vi "AuMT8852B Single-slot Sensitivity Configuration.vi"(5 "Settings":T1={"Low frequency selection"=enum."Use low frequency", "Medium frequency selection"=enum."Use medium frequency", "High frequency selection"=enum."Use high frequency", "Low TX frequency"=2480.0, "Low RX frequency"=2402.0, "Medium TX frequency"=2402.0, "Medium RX frequency"=2441.0, "High TX frequency"=2402.0, "High RX frequency"=2480.0, "Number of packets"=7408, "Test TX power"=-70.0, "BER limit"=0.1, "FER limit"=100.0, "Hop selection"=enum."Test with hopping off and on", "Packet count"=enum."TX", "Use Dirty transmitter"=FALSE, "Frequency offset (kHz)"=[75.0, 14.0, -2.0, 1.0, 39.0, 0.0, -42.0, 74.0, -19.0, -75.0], "Symbol timing error (ppm)"=[-20.0, -20.0, 20.0, 20.0, 20.0, -20.0, -20.0, -20.0, -20.0, 20.0], "Modulation index"=[0.28, 0.3, 0.29, 0.32, 0.33, 0.34, 0.29, 0.31, 0.28, 0.35]} {"Frequency offset (kHz)" format="%.2f"; "Symbol timing error (ppm)" format="%.2f"; "FER limit" format="%.2f"; "BER limit" format="%.2f"; "Modulation index" format="%.2f"; "Test TX power" format="%.1f"}, 7 "Set/Get (Set)":enum16{"Set", "Get"}(ring), 8 "error in (no error)":errorcluster, 10 "Script (3)":i32=3, 11 "VISA session":refnum<visa-resource-name>) -> (0 "error out":errorcluster, 2 "error code":i32, 3 "VISA session out":refnum<visa-resource-name>, 4 "Settings out":T1={"Low frequency selection"=enum."Use low frequency", "Medium frequency selection"=enum."Use medium frequency", "High frequency selection"=enum."Use high frequency", "Low TX frequency"=0.0, "Low RX frequency"=0.0, "Medium TX frequency"=0.0, "Medium RX frequency"=0.0, "High TX frequency"=0.0, "High RX frequency"=0.0, "Number of packets"=0, "Test TX power"=0.0, "BER limit"=0.0, "FER limit"=0.0, "Hop selection"=enum."Test with hopping on", "Packet count"=enum."TX", "Use Dirty transmitter"=FALSE, "Frequency offset (kHz)"=[], "Symbol timing error (ppm)"=[], "Modulation index"=[]} {"Symbol timing error (ppm)" format="%.2f"; "Modulation index" format="%.2f"; "Frequency offset (kHz)" format="%.2f"; "FER limit" format="%.2f"; "BER limit" format="%.2f"; "Test TX power" format="%.1f"})   [LabVIEW 2017]
doc: "Anritsu MT8852B Bluetooth Tester\n\nConfigures the instrument for the Single-slot Sensitivity test.\n\nINPUTS\nSet/Get - whether the values are being sent to or retrieved from the instrument.\nScript - which of the stored scripts (1-10) will be queried or configured. Scripts 1 and 2 are read-only.\nSettings - parameters of the test to be written.\n\nOUTPUTS\nSettings out - current parameters of the test."
uses:
  <instrlib>/aumt8852B/General/Utilities/MT8850 Test Parameters.ctl
  <instrlib>/aumt8852B/General/Utilities/MT8850 Frequency Units.ctl
panel:
  in  "Case Constant\n(See Context Help)":bool
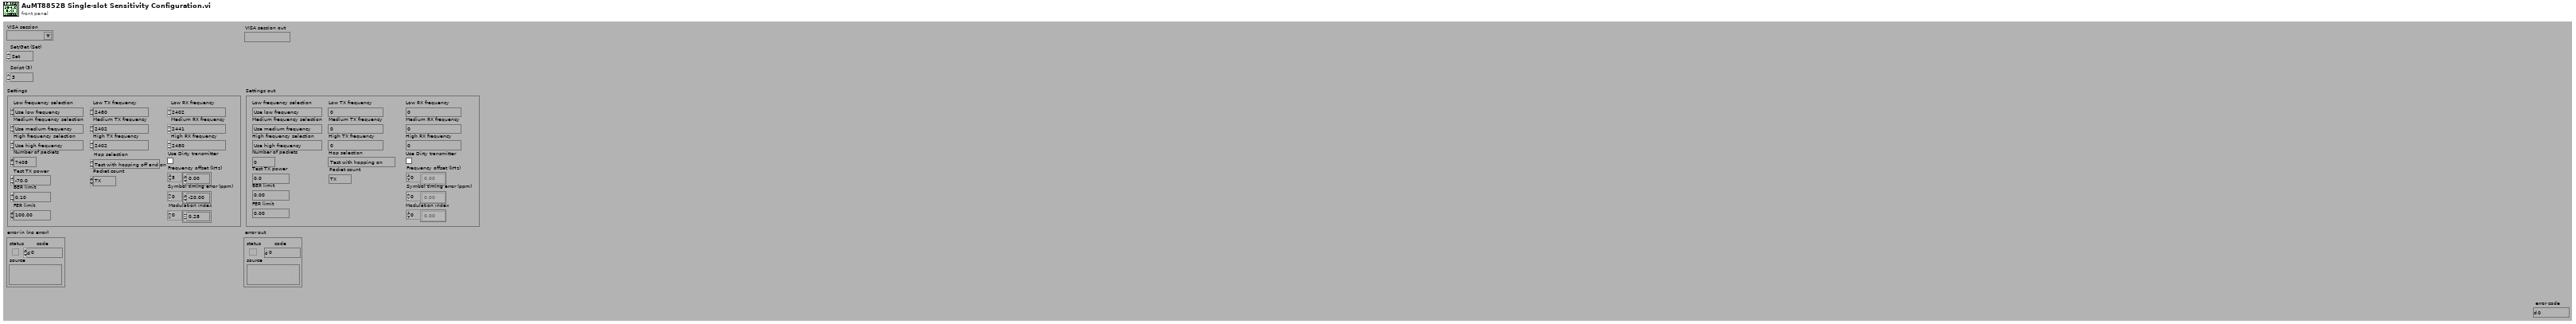
[diagram p1: front panel]
types:
  T1 = cluster{"Low frequency selection":enum16{"Don't use low frequency", "Use low frequency"}, "Medium frequency selection":enum16{"Don't use medium frequency", "Use medium frequency"}, "High frequency selection":enum16{"Don't use high frequency", "Use high frequency"}, "Low TX frequency":dbl, "Low RX frequency":dbl, "Medium TX frequency":dbl, "Medium RX frequency":dbl, "High TX frequency":dbl, "High RX frequency":dbl, "Number of packets":i32, "Test TX power":dbl, "BER limit":dbl, "FER limit":dbl, "Hop selection":enum16{"Test with hopping on", "Test with hopping off", "Test with hopping off and on"}, "Packet count":enum16{"TX", "RX"}, "Use Dirty transmitter":bool, "Frequency offset (kHz)":dbl[], "Symbol timing error (ppm)":dbl[], "Modulation index":dbl[]}
  T2 = typedef "MT8850 Test Parameters.ctl" = enum16{"Use low frequency", "Use medium frequency", "Use high frequency", "Low TX frequency", "Low RX frquency", "Medium TX frequency", "Medium RX frequency", "High TX frequency", "High RX frequency", "Number of packets", "Average high limit", "Average low limit", "Peak power limit", "Max power step limit", "Min power step limit", "f1 average minimum", "f1 average maximum", "f2 maximum", "f1/f2 average maximum", "Hop selection", "Use DH1 packets", "Use DH3 packets", "Use DH5 packets", "1 slot packet drift limit", "3 slot packet drift limit", "5 slot packet drift limit", "Drift rate limit", "TX power level", "Frequency offset", "Symbol timing", "Modulation index", "BER limit", "FER limit", "Use averaging high limit", "Use averaging low limit", "Use peak power limit", "Packet type", "Test control", "Use max power step limit", "Use min power step limit", "Number of cycles", "Use f1 average maximum", "Use f1 average minimum", "Use f2 maximum", "Use f1/f2 average maximum", "Hop mode", "Maximum negative limit", "Maximum positive limit", "Use maximum negative limit", "Use maximum positive limit", "Use 1 slot packet drift limit", "Use 3 slot packet drift limit", "Use 5 slot packet drift limit", "Use drift rate limit", "Use BER limit", "Use FER limit", "Use dirty parameter table", "Use null packet drift limit", "Null packet drift limit", "Minimum power", "Power delay", "Packet count", "Payload toggle", "Output power level", "2DHX packet type", "3DHX packet type", "Number of blocks", "TX and RX low frequency", "TX and RX medium frequency", "TX and RX high frequency", "TX frequency", "RX frequency", "Threshold bit count", "Total test bit count", "Number of bits", "PDPSK to PGFSK lower limit", "PDPSK to PGFSK upper limit", "Initial frequency error upper limit", "Initial frequency error lower limit", "Frequency error upper limit", "Frequency error lower limit", "Block frequency error upper limit", "Block frequency error lower limit", "2Mbs RMS DEVM limit", "3Mbs RMS DEVM limit", "2Mbs Peak DEVM limit", "3Mbs Peak DEVM limit", "2Mbs 99% packets DEVM limit", "3Mbs 99% packets DEVM limit", "Percentage of no error packets limit", "Threshold error limit", "Total test error limit"}
  T3 = enum16{"Single-slot sensitivity", "Multiple-slot sensitivity"}
  T4 = enum16{"Frequency offset", "Symbol timing value", "Mod index value"}
  T5 = typedef "MT8850 Frequency Units.ctl" = enum16{"Channel", "Hz", "kHz", "MHz", "GHz"}
  T6 = enum16{"Simulate", "Range check", "Cache", "Query instrument status"}
  T7 = enum16{"Output power", "Power control", "Modulation characteristics", "Initial carrier", "Carrier drift", "Single slot sensitivity", "Multiple slot sensitivity", "Maximum input power"}
  T8 = enum16{"Test with hopping on", "Test with hopping off", "Test with hopping off and on"}
  T9 = enum16{"Don't use high frequency", "Use high frequency"}
  T10 = enum16{"Don't use medium frequency", "Use medium frequency"}
  T11 = enum16{"Don't use low frequency", "Use low frequency"}
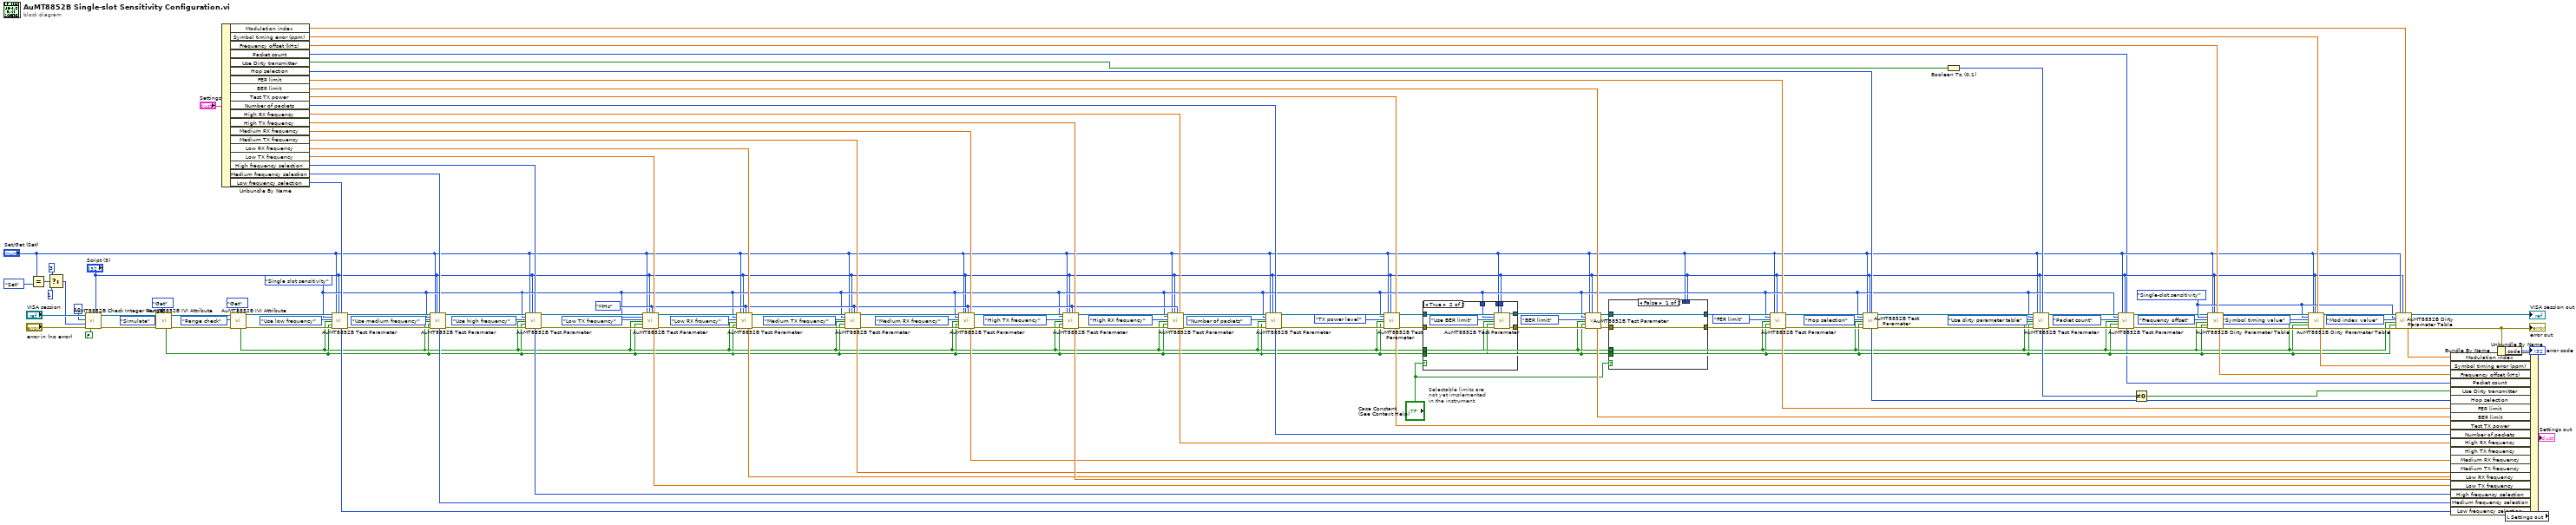
[diagram p0: block diagram]
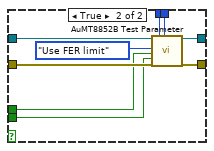
[diagram p2: hidden frame]
diagram:
  w13 = T3."Single-slot sensitivity" ("Test (Single-slot sensitivity)")
  w35 = MT8850_Frequency_Units."MHz" ("Frequency units (MHz)")
  w8 = T7."Single slot sensitivity" ("Test (Output Power)")
  # "Selectable limits are\nnot yet implemented\nin the instrument."
  n1 = Equal?(x="Set/Get (Set)", y=enum16{"Set", "Get"}."Set") -> (x = y?=w129:bool)
  n2 = Select(t=3, s=w129, f=1) -> (s? t:f=w125:i32)
  n3 = call <instrlib>:"AuMT8852B Check Integer Range.vi"("Value (0)"="Script (3)", "Check IVI flag first? (T)"=FALSE, "error in (no error)"="error in (no error)", "Lower limit (-1)"=w125, "Upper limit (1)"=10, "VISA session"="VISA session") -> ("error out"=w123:errorcluster, "VISA session out"=w124:refnum<visa-resource-name>)  [unwired: 4 in]
  n4 = call <instrlib>:"AuMT8852B IVI Attribute.vi"("Set/Get (Set)"=enum16{"Set", "Get"}."Get", "error in (no error)"=w123, "Flag (Simulate)"=T6."Simulate", "VISA session"=w124) -> ("error out"=w97:errorcluster, "VISA session out"=w98:refnum<visa-resource-name>, "Value out"=w3:bool)  [unwired: 5 in]
  n5 = Unbundle By Name("Settings") -> ("Modulation index"=w24:dbl[], "Symbol timing error (ppm)"=w25:dbl[], "Frequency offset (kHz)"=w29:dbl[], "Packet count"=w1:enum16{"TX", "RX"}, "Use Dirty transmitter"=w47:bool, "Hop selection"=w51:T8, "FER limit"=w65:dbl, "BER limit"=w66:dbl, "Test TX power"=w70:dbl, "Number of packets"=w71:i32, "High RX frequency"=w84:dbl, "High TX frequency"=w85:dbl, "Medium RX frequency"=w72:dbl, "Medium TX frequency"=w86:dbl, "Low RX frequency"=w87:dbl, "Low TX frequency"=w88:dbl, "High frequency selection"=w89:T9, "Medium frequency selection"=w90:T10, "Low frequency selection"=w91:T11)
  n6 = call <instrlib>:"AuMT8852B IVI Attribute.vi"("Set/Get (Set)"=enum16{"Set", "Get"}."Get", "error in (no error)"=w97, "Flag (Simulate)"=T6."Range check", "VISA session"=w98) -> ("error out"=w95:errorcluster, "VISA session out"=w96:refnum<visa-resource-name>, "Value out"=w4:bool)  [unwired: 5 in]
  n7 = call <instrlib>:"AuMT8852B Test Parameter.vi"("VISA session"=w96, "Test (Output power)"=w8, "Parameter (Use low frequency)"=MT8850_Test_Parameters."Use low frequency", "Range check? (F)"=w4, "Simulate? (F)"=w3, "error in (no error)"=w95, "Set/Get (Set)"="Set/Get (Set)", "Script (3)"="Script (3)", "Integer value (0)"=w91) -> ("Integer value out"=w76:i32, "VISA session out"=w43:refnum<visa-resource-name>, "error out"=w42:errorcluster)  [unwired: 7 in, 1 out]
  n8 = call <instrlib>:"AuMT8852B Test Parameter.vi"("VISA session"=w43, "Test (Output power)"=w8, "Parameter (Use low frequency)"=MT8850_Test_Parameters."Use medium frequency", "Range check? (F)"=w4, "Simulate? (F)"=w3, "error in (no error)"=w42, "Set/Get (Set)"="Set/Get (Set)", "Script (3)"="Script (3)", "Integer value (0)"=w90) -> ("Integer value out"=w77:i32, "VISA session out"=w41:refnum<visa-resource-name>, "error out"=w40:errorcluster)  [unwired: 7 in, 1 out]
  n9 = call <instrlib>:"AuMT8852B Test Parameter.vi"("VISA session"=w41, "Test (Output power)"=w8, "Parameter (Use low frequency)"=MT8850_Test_Parameters."Use high frequency", "Range check? (F)"=w4, "Simulate? (F)"=w3, "error in (no error)"=w40, "Set/Get (Set)"="Set/Get (Set)", "Script (3)"="Script (3)", "Integer value (0)"=w89) -> ("Integer value out"=w78:i32, "VISA session out"=w119:refnum<visa-resource-name>, "error out"=w118:errorcluster)  [unwired: 7 in, 1 out]
  n10 = call <instrlib>:"AuMT8852B Test Parameter.vi"("VISA session"=w119, "Test (Output power)"=w8, "Parameter (Use low frequency)"=MT8850_Test_Parameters."Low TX frequency", "Range check? (F)"=w4, "Simulate? (F)"=w3, "error in (no error)"=w118, "Set/Get (Set)"="Set/Get (Set)", "Script (3)"="Script (3)", "Integer value (0)"=w35, "Float value (0)"=w88) -> ("Float value out"=w79:dbl, "VISA session out"=w117:refnum<visa-resource-name>, "error out"=w116:errorcluster)  [unwired: 6 in, 1 out]
  n11 = call <instrlib>:"AuMT8852B Test Parameter.vi"("VISA session"=w117, "Test (Output power)"=w8, "Parameter (Use low frequency)"=MT8850_Test_Parameters."Low RX frquency", "Range check? (F)"=w4, "Simulate? (F)"=w3, "error in (no error)"=w116, "Set/Get (Set)"="Set/Get (Set)", "Script (3)"="Script (3)", "Integer value (0)"=w35, "Float value (0)"=w87) -> ("Float value out"=w80:dbl, "VISA session out"=w115:refnum<visa-resource-name>, "error out"=w114:errorcluster)  [unwired: 6 in, 1 out]
  n12 = call <instrlib>:"AuMT8852B Test Parameter.vi"("VISA session"=w115, "Test (Output power)"=w8, "Parameter (Use low frequency)"=MT8850_Test_Parameters."Medium TX frequency", "Range check? (F)"=w4, "Simulate? (F)"=w3, "error in (no error)"=w114, "Set/Get (Set)"="Set/Get (Set)", "Script (3)"="Script (3)", "Integer value (0)"=w35, "Float value (0)"=w86) -> ("Float value out"=w81:dbl, "VISA session out"=w113:refnum<visa-resource-name>, "error out"=w112:errorcluster)  [unwired: 6 in, 1 out]
  n13 = call <instrlib>:"AuMT8852B Test Parameter.vi"("VISA session"=w113, "Test (Output power)"=w8, "Parameter (Use low frequency)"=MT8850_Test_Parameters."Medium RX frequency", "Range check? (F)"=w4, "Simulate? (F)"=w3, "error in (no error)"=w112, "Set/Get (Set)"="Set/Get (Set)", "Script (3)"="Script (3)", "Integer value (0)"=w35, "Float value (0)"=w72) -> ("Float value out"=w74:dbl, "VISA session out"=w111:refnum<visa-resource-name>, "error out"=w110:errorcluster)  [unwired: 6 in, 1 out]
  n14 = call <instrlib>:"AuMT8852B Test Parameter.vi"("VISA session"=w111, "Test (Output power)"=w8, "Parameter (Use low frequency)"=MT8850_Test_Parameters."High TX frequency", "Range check? (F)"=w4, "Simulate? (F)"=w3, "error in (no error)"=w110, "Set/Get (Set)"="Set/Get (Set)", "Script (3)"="Script (3)", "Integer value (0)"=w35, "Float value (0)"=w85) -> ("Float value out"=w82:dbl, "VISA session out"=w109:refnum<visa-resource-name>, "error out"=w108:errorcluster)  [unwired: 6 in, 1 out]
  n15 = call <instrlib>:"AuMT8852B Test Parameter.vi"("VISA session"=w109, "Test (Output power)"=w8, "Parameter (Use low frequency)"=MT8850_Test_Parameters."High RX frequency", "Range check? (F)"=w4, "Simulate? (F)"=w3, "error in (no error)"=w108, "Set/Get (Set)"="Set/Get (Set)", "Script (3)"="Script (3)", "Integer value (0)"=w35, "Float value (0)"=w84) -> ("Float value out"=w83:dbl, "VISA session out"=w107:refnum<visa-resource-name>, "error out"=w106:errorcluster)  [unwired: 6 in, 1 out]
  n16 = call <instrlib>:"AuMT8852B Test Parameter.vi"("VISA session"=w107, "Test (Output power)"=w8, "Parameter (Use low frequency)"=MT8850_Test_Parameters."Number of packets", "Range check? (F)"=w4, "Simulate? (F)"=w3, "error in (no error)"=w106, "Set/Get (Set)"="Set/Get (Set)", "Script (3)"="Script (3)", "Integer value (0)"=w71) -> ("Integer value out"=w73:i32, "VISA session out"=w34:refnum<visa-resource-name>, "error out"=w33:errorcluster)  [unwired: 7 in, 1 out]
  n17 = call <instrlib>:"AuMT8852B Test Parameter.vi"("VISA session"=w34, "Test (Output power)"=w8, "Parameter (Use low frequency)"=MT8850_Test_Parameters."TX power level", "Range check? (F)"=w4, "Simulate? (F)"=w3, "error in (no error)"=w33, "Set/Get (Set)"="Set/Get (Set)", "Script (3)"="Script (3)", "Float value (0)"=w70) -> ("Float value out"=w64:dbl, "VISA session out"=w22:refnum<visa-resource-name>, "error out"=w23:errorcluster)  [unwired: 7 in, 1 out]
  n18 = case shown="True" "Case Constant\n(See Context Help)" {
    tunnel: w23 -> [w133 w143]
    tunnel: w22 -> [w134 w142]
    tunnel: [w134 w141] -> w57
    tunnel: [w133 w140] -> w56
    tunnel: w8 -> [_ w139]
    tunnel: w4 -> [_ w138]
    tunnel: w3 -> [_ w137]
    tunnel: "Set/Get (Set)" -> [_ w136]
    tunnel: "Script (3)" -> [_ w135]
    frame False {
    }
    frame True {
      n19 = call <instrlib>:"AuMT8852B Test Parameter.vi"("VISA session"=w142, "Test (Output power)"=w139, "Parameter (Use low frequency)"=MT8850_Test_Parameters."Use BER limit", "Range check? (F)"=w138, "Simulate? (F)"=w137, "error in (no error)"=w143, "Set/Get (Set)"=w136, "Script (3)"=w135) -> ("VISA session out"=w141:refnum<visa-resource-name>, "error out"=w140:errorcluster)  [unwired: 8 in, 2 out]
    }
  }
  n20 = call <instrlib>:"AuMT8852B Test Parameter.vi"("VISA session"=w57, "Test (Output power)"=w8, "Parameter (Use low frequency)"=MT8850_Test_Parameters."BER limit", "Range check? (F)"=w4, "Simulate? (F)"=w3, "error in (no error)"=w56, "Set/Get (Set)"="Set/Get (Set)", "Script (3)"="Script (3)", "Float value (0)"=w66) -> ("Float value out"=w63:dbl, "VISA session out"=w54:refnum<visa-resource-name>, "error out"=w55:errorcluster)  [unwired: 7 in, 1 out]
  n21 = case shown="False" "Case Constant\n(See Context Help)" {
    tunnel: w55 -> [w145 w154]
    tunnel: w54 -> [w146 w153]
    tunnel: [w146 w152] -> w53
    tunnel: [w145 w151] -> w52
    tunnel: w4 -> [_ w150]
    tunnel: w3 -> [_ w149]
    tunnel: "Set/Get (Set)" -> [_ w148]
    tunnel: "Script (3)" -> [_ w147]
    frame False {
    }
    frame True {
      n22 = call <instrlib>:"AuMT8852B Test Parameter.vi"("VISA session"=w153, "Parameter (Use low frequency)"=MT8850_Test_Parameters."Use FER limit", "Range check? (F)"=w150, "Simulate? (F)"=w149, "error in (no error)"=w154, "Set/Get (Set)"=w148, "Script (3)"=w147) -> ("VISA session out"=w152:refnum<visa-resource-name>, "error out"=w151:errorcluster)  [unwired: 9 in, 2 out]
    }
  }
  n23 = call <instrlib>:"AuMT8852B Test Parameter.vi"("VISA session"=w53, "Test (Output power)"=w8, "Parameter (Use low frequency)"=MT8850_Test_Parameters."FER limit", "Range check? (F)"=w4, "Simulate? (F)"=w3, "error in (no error)"=w52, "Set/Get (Set)"="Set/Get (Set)", "Script (3)"="Script (3)", "Float value (0)"=w65) -> ("Float value out"=w62:dbl, "VISA session out"=w59:refnum<visa-resource-name>, "error out"=w60:errorcluster)  [unwired: 7 in, 1 out]
  n24 = call <instrlib>:"AuMT8852B Test Parameter.vi"("VISA session"=w59, "Test (Output power)"=w8, "Parameter (Use low frequency)"=MT8850_Test_Parameters."Hop selection", "Range check? (F)"=w4, "Simulate? (F)"=w3, "error in (no error)"=w60, "Set/Get (Set)"="Set/Get (Set)", "Script (3)"="Script (3)", "Integer value (0)"=w51) -> ("Integer value out"=w58:i32, "VISA session out"=w32:refnum<visa-resource-name>, "error out"=w31:errorcluster)  [unwired: 7 in, 1 out]
  n25 = Boolean To (0,1)(Boolean=w47) -> (0, 1=w48:i16)
  n26 = call <instrlib>:"AuMT8852B Test Parameter.vi"("VISA session"=w32, "Test (Output power)"=w8, "Parameter (Use low frequency)"=MT8850_Test_Parameters."Use dirty parameter table", "Range check? (F)"=w4, "Simulate? (F)"=w3, "error in (no error)"=w31, "Set/Get (Set)"="Set/Get (Set)", "Script (3)"="Script (3)", "Integer value (0)"=w48) -> ("Integer value out"=w49:i32, "VISA session out"=w12:refnum<visa-resource-name>, "error out"=w11:errorcluster)  [unwired: 7 in, 1 out]
  n27 = call <instrlib>:"AuMT8852B Test Parameter.vi"("VISA session"=w12, "Test (Output power)"=w8, "Parameter (Use low frequency)"=MT8850_Test_Parameters."Packet count", "Range check? (F)"=w4, "Simulate? (F)"=w3, "error in (no error)"=w11, "Set/Get (Set)"="Set/Get (Set)", "Script (3)"="Script (3)", "Integer value (0)"=w1) -> ("Integer value out"=w2:i32, "VISA session out"=w9:refnum<visa-resource-name>, "error out"=w10:errorcluster)  [unwired: 7 in, 1 out]
  n28 = Not Equal To 0?(x=w49) -> (x != 0?=w50:bool)
  n29 = call <instrlib>:"AuMT8852B Dirty Parameter Table.vi"("VISA session"=w9, "Test (Single-slot sensitivity)"=w13, "Variable (Frequency offset)"=T4."Frequency offset", "Range check? (F)"=w4, "Simulate? (F)"=w3, "error in (no error)"=w10, "Set/Get (Set)"="Set/Get (Set)", "Script (3)"="Script (3)", "Parameters"=w29) -> ("Parameters out"=w28:dbl[], "VISA session out"=w19:refnum<visa-resource-name>, "error out"=w18:errorcluster)  [unwired: 8 in]
  n30 = call <instrlib>:"AuMT8852B Dirty Parameter Table.vi"("VISA session"=w19, "Test (Single-slot sensitivity)"=w13, "Variable (Frequency offset)"=T4."Symbol timing value", "Range check? (F)"=w4, "Simulate? (F)"=w3, "error in (no error)"=w18, "Set/Get (Set)"="Set/Get (Set)", "Script (3)"="Script (3)", "Parameters"=w25) -> ("Parameters out"=w27:dbl[], "VISA session out"=w17:refnum<visa-resource-name>, "error out"=w16:errorcluster)  [unwired: 8 in]
  n31 = call <instrlib>:"AuMT8852B Dirty Parameter Table.vi"("VISA session"=w17, "Test (Single-slot sensitivity)"=w13, "Variable (Frequency offset)"=T4."Mod index value", "Range check? (F)"=w4, "Simulate? (F)"=w3, "error in (no error)"=w16, "Set/Get (Set)"="Set/Get (Set)", "Script (3)"="Script (3)", "Parameters"=w24) -> ("Parameters out"=w26:dbl[], "VISA session out"=→"VISA session out":refnum<visa-resource-name>, "error out"=w36:errorcluster)  [unwired: 8 in]
  "error out" <- w36
  n32 = Unbundle By Name(w36) -> ("code"=→"error code":i32)
  n33 = local read "Settings out"() -> (w75:T1)
  n34 = Bundle By Name(cluster=w75, "Modulation index"=w26, "Symbol timing error (ppm)"=w27, "Frequency offset (kHz)"=w28, "Packet count"=w2, "Use Dirty transmitter"=w50, "Hop selection"=w58, "FER limit"=w62, "BER limit"=w63, "Test TX power"=w64, "Number of packets"=w73, "High RX frequency"=w83, "High TX frequency"=w82, "Medium RX frequency"=w74, "Medium TX frequency"=w81, "Low RX frequency"=w80, "Low TX frequency"=w79, "High frequency selection"=w78, "Medium frequency selection"=w77, "Low frequency selection"=w76) -> (→"Settings out":T1)
